vi "get value from cmd array.vi"(10 "element":string, 11 "cmds":string[](array[string])) -> (2 "valid?":bool, 3 "value":string)   [LabVIEW 2020]
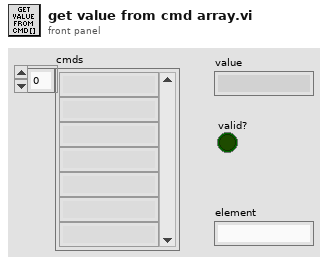
[diagram p1: front panel]
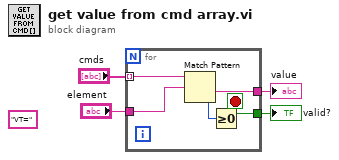
[diagram p0: block diagram]
diagram:
  (unwired) "VT=" ("regular expression")
  n1 = for {
    tunnel: "cmds" -> [w9] mode=indexing
    tunnel: [w8] -> w3
    tunnel: [w6] -> w4
    tunnel: "element" -> [w5]
    stop <- w6 stop-if-true
    n2 = Match Pattern(string=w9, regular expression=w5) -> (after substring=w8:string, offset past match=w7:i32)  [unwired: 1 in, 2 out]
    n3 = Greater Or Equal To 0?(x=w7) -> (x >= 0?=w6:bool)
  }
  "valid?" <- w4
  "value" <- w3
